vi "SerializePrivateControl.vi"(7 "App Ref":refnum<vi>, 8 "error in (no error)":errorcluster, 9 "Output JSON File Path":path, 10 "Library":refnum<vi>, 11 "Root in":refnum<data-value>) -> (0 "error out":errorcluster, 3 "Root out":refnum<data-value>)   [LabVIEW 2017, in "ClassConverter.lvclass"]
uses:
  ClassConverter.lvclass
  Helpers/DirectoryMetadata/DirectoryMetadata.lvclass
  VIConverter/VIConverter.lvclass
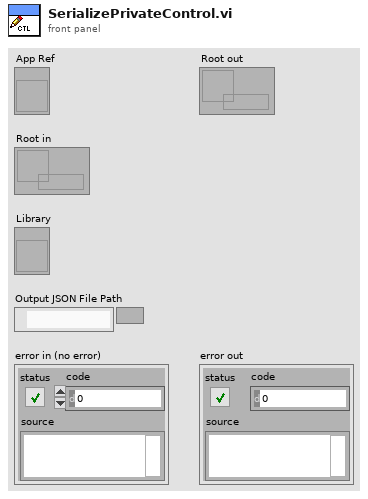
[diagram p1: front panel]
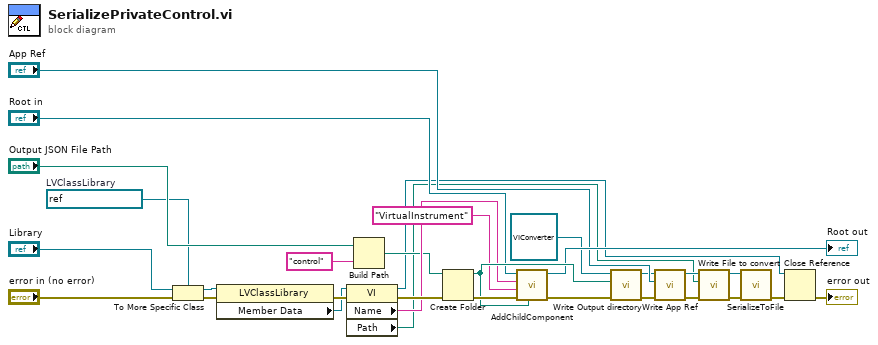
[diagram p0: block diagram]
diagram:
  w7 = refnum<vi> refnum  # LVClassLibrary
  n1 = To More Specific Class(target class=w7, reference="Library", error in="error in (no error)") -> (specific class reference=w6:refnum<vi>, error out=w8:errorcluster)
  n2 = property class="LVClassLibrary"(reference=w6, error in=w8) -> (error out=w26:errorcluster, "Member Data"=w21:refnum<vi>)  [unwired: 1 out]
  n3 = property class="VI"(reference=w21, error in=w26) -> (reference out=w1:refnum<vi>, error out=w28:errorcluster, "Name"=w22:string, "Path"=w3:path)
  n4 = Build Path(base path="Output JSON File Path", name or relative path="control") -> (appended path=w11:path)
  n5 = Create Folder(path (use dialog)=w11, error in=w28) -> (created path=w27:path, error out=w29:errorcluster)  [unwired: 1 in, 1 out]
  n6 = call "AddChildComponent.vi"("Path"=w27, "error in (no error)"=w29, "Type"="VirtualInstrument", "ID"=w22, "head in"="Root in") -> ("error out"=w30:errorcluster, "head out"=→"Root out":refnum<data-value>)  [unwired: 4 in, 1 out]
  n7 = call-dynamic "Write Output directory.vi"("error in (no error)"=w30, "Output JSON File Path"=w27, "FileConverterBase in"=refnum<class "VIConverter.lvclass"> refnum ("VIConverter.lvclass")) -> ("error out"=w18:errorcluster, "FileConverterBase out"=w15:refnum<class "VIConverter.lvclass">)  [unwired: 7 in]
  n8 = call-dynamic "Write App Ref.vi"("error in (no error)"=w18, "App Ref"="App Ref", "FileConverterBase in"=w15) -> ("error out"=w2:errorcluster, "FileConverterBase out"=w16:refnum<class "VIConverter.lvclass">)  [unwired: 7 in]
  n9 = call-dynamic "Write File to convert.vi"("error in (no error)"=w2, "Input File Path"=w3, "FileConverterBase in"=w16) -> ("error out"=w13:errorcluster, "FileConverterBase out"=w14:refnum<class "VIConverter.lvclass">)  [unwired: 7 in]
  n10 = call-dynamic "SerializeToFile.vi"("error in (no error)"=w13, "FileConverterBase in"=w14) -> ("error out"=w4:errorcluster)  [unwired: 8 in, 1 out]
  n11 = Close Reference(reference=w1, error in (no error)=w4) -> (error out=→"error out":errorcluster)
